vi "Find Com Port by Model.vi"(9 "Array":T1[](array[typedef]), 11 "Power Supply Serial Number":string="6474001050") -> (3 "String":string)   [LabVIEW 2015]
uses:
  Resource Data.ctl
panel:
  out "Found":bool
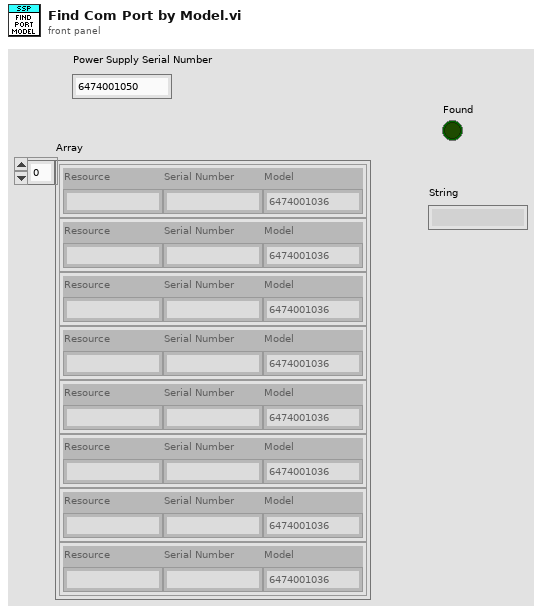
[diagram p1: front panel]
types:
  T1 = typedef "Resource Data.ctl" = cluster{"Resource":string, "Serial Number":string, "Model":string}
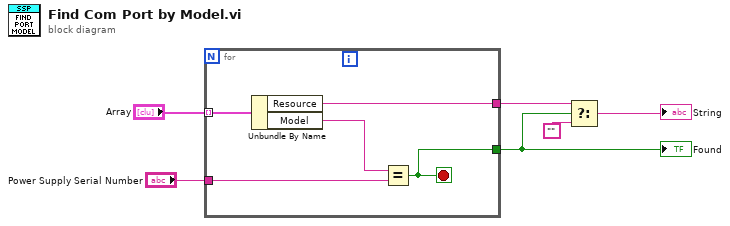
[diagram p0: block diagram]
diagram:
  n1 = for {
    tunnel: "Array" -> [w10] mode=indexing
    tunnel: "Power Supply Serial Number" -> [w8]
    tunnel: [w11] -> w5
    tunnel: [w7] -> w2
    stop <- w11 stop-if-true
    n2 = Unbundle By Name(w10) -> ("Resource"=w7:string, "Model"=w9:string)
    n3 = Equal?(x=w9, y=w8) -> (x = y?=w11:bool)
  }
  "Found" <- w5
  n4 = Select(t=w2, s=w5, f="") -> (s? t:f=→"String":string)
